vi "接收字符串截取功能.vi"(11 "输入结果":string) -> (0 "输出结果":string, 3 "工位名称":string)   [LabVIEW 2011]
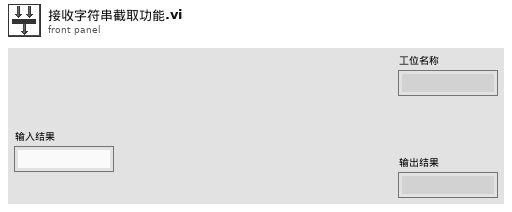
[diagram p1: front panel]
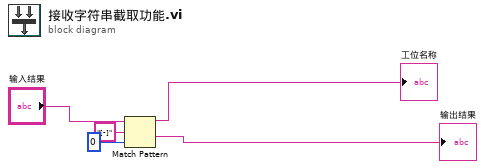
[diagram p0: block diagram]
diagram:
  n1 = Match Pattern(string="输入结果", regular expression="[-]" ("正则表达式"), offset (0)=0 ("偏移量(0)")) -> (before substring=→"工位名称":string, after substring=→"输出结果":string)  [unwired: 2 out]
